vi "SE FP behavior point to dock.vi"(1 "GPS":cluster{"X pos":i32, "Y pos":i32, "Heading":dbl}, 2 "IR Sensors":T1(array[cluster]), 3 "GPS Initial":cluster{"X pos":i32, "Y pos":i32, "Heading":dbl}, 4 "Behavior\nVelocity":dbl, 5 "Activate?":bool=TRUE, 6 "Camera Data":T2(array[cluster])) -> (0 "Dock Array":dbl[](array[numeric]))   [LabVIEW 2014]
panel:
  out "Waveform Graph":cluster{dbl, dbl, dbl[]}(graph)
  # "Dock"
  # "Current"
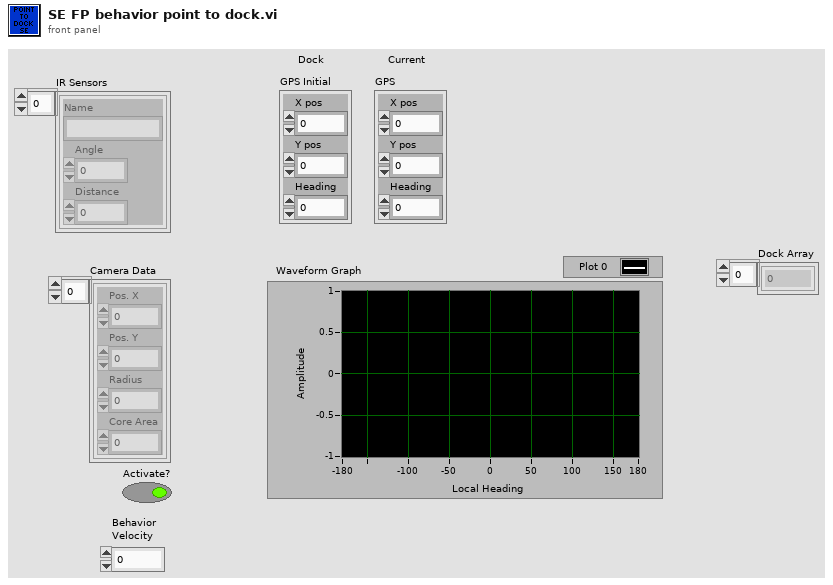
[diagram p1: front panel]
types:
  T1 = cluster{"Name":string, "Angle":dbl, "Distance":dbl}[]
  T2 = cluster{"Pos. X":i32, "Pos. Y":i32, "Radius":i32, "Core Area":i32}[]
  T3 = cluster{"Name":string, "Angle":dbl, "Distance":dbl}
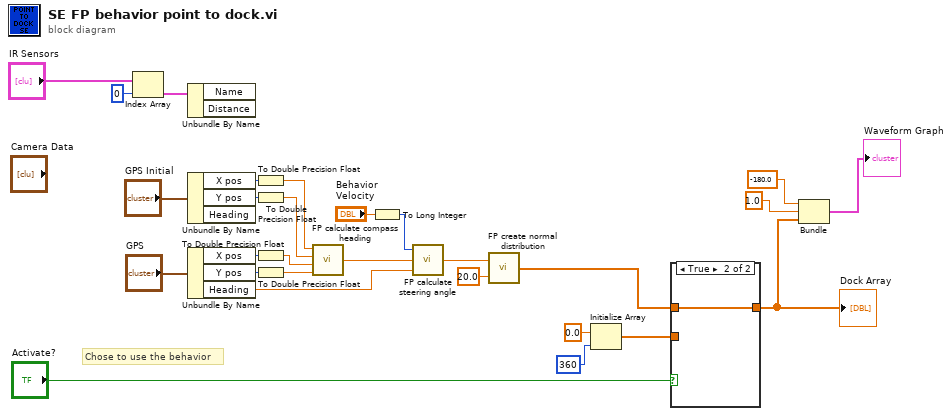
[diagram p0: block diagram]
diagram:
  # "Chose to use the behavior"
  n1 = Index Array(array="IR Sensors", index=0) -> (element=w19:T3)
  n2 = Unbundle By Name(w19) -> ()  [unwired: 2 out]
  n3 = Unbundle By Name("GPS Initial") -> ("X pos"=w11:i32, "Y pos"=w10:i32)  [unwired: 1 out]
  n4 = Unbundle By Name("GPS") -> ("X pos"=w15:i32, "Y pos"=w14:i32, "Heading"=w6:dbl)
  n5 = To Double Precision Float(number=w11) -> (double precision float=w9:dbl)
  n6 = To Double Precision Float(number=w10) -> (double precision float=w8:dbl)
  n7 = To Double Precision Float(number=w15) -> (double precision float=w13:dbl)
  n8 = To Double Precision Float(number=w14) -> (double precision float=w12:dbl)
  n9 = call "FP calculate compass heading.vi"("Y Location"=w12, "X Location"=w13, "Waypoint Y"=w8, "Waypoint X"=w9) -> ("Heading"=w7:dbl)
  n10 = To Long Integer(number="Behavior\nVelocity") -> (32bit integer=w4:i32)
  n11 = call "FP calculate steering angle.vi"("Compass\nheading"=w6, "New heading"=w7, "Speed"=w4) -> ("Local Steering Angle"=w3:dbl)
  n12 = call "FP create normal distribution.vi"("std (Normal)"=20.0, "mean"=w3) -> ("ACT array"=w1:dbl[])
  n13 = Initialize Array(0.0 ("element"), 360 ("dimension size")) -> (w22:dbl[])
  n14 = case shown="True" "Activate?" {
    tunnel: w22 -> [w29 _]
    tunnel: w1 -> [_ w30]
    tunnel: [w29 w30] -> w21
    frame False {
    }
    frame True {
    }
  }
  "Dock Array" <- w21
  n15 = Bundle(-180.0, 1.0, "ACT array"=w21) -> (→"Waveform Graph":cluster{dbl, dbl, "ACT array":dbl[]})  [unwired: 1 in]
